vi "Read.vi"(7 "I2C Channel":u8, 8 "Error In":errorcluster, 9 "Range Magnitude (g's)":u16=2, 10 "I2C Slave Address (0x1D)":u8, 11 "LINX Resource in":T1) -> (0 "Error Out":errorcluster, 2 "Acceleration Data (g)":T7, 3 "LINX Resource out":T1)   [LabVIEW 2020, in "LMH-LINX.lvlib" / "MMA8452.lvlib"]
uses:
  MMA8452.lvlib
  Private/Type Defs/LINX Ref.ctl
  Private/Type Defs/Platform.ctl
  Private/Type Defs/Interface.ctl
  Private/Device/Type Defs/LINX Device Config.ctl
  Private/Device/Type Defs/TCP Config.ctl
  Private/Device/Type Defs/Channels.ctl
  Private/Type Defs/Peripherals/I2C/EOF.ctl
  Private/Local IO/LinxI2cWrite.vi
  Utilities/Check Channel.vi
  Private/Utilties/Generate Error.vi
  LMH-LINX.lvlib
  Toolbox/LMH-Toolbox.lvlib
  Private/Device/Device.lvlib
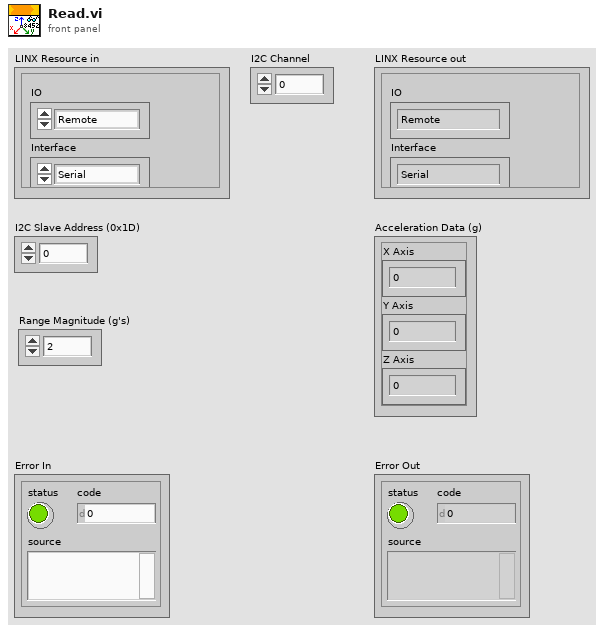
[diagram p1: front panel]
types:
  T1 = typedef "LMH-LINX.lvlib/LINX Ref.ctl" = cluster{"IO":T2, "Interface":T3, "LINX Device Config":T4}
  T2 = typedef "LMH-LINX.lvlib/Platform.ctl" = enum16{"Remote", "Local"}
  T3 = typedef "LMH-LINX.lvlib/Interface.ctl" = enum16{"Serial", "TCP"}
  T4 = typedef "Device.lvlib/LINX Device Config.ctl" = cluster{"Interface":T3, "COM Port":refnum<visa-resource-name>, "TCP Configuration":T5, "Device Family":u8, "Device ID":u8, "Device Name":string, "TCP Ref":refnum<k5>, "Channels":T6}
  T5 = typedef "Device.lvlib/TCP Config.ctl" = cluster{"IP Address":string, "Port":u16}
  T6 = typedef "LMH-LINX.lvlib/Channels.ctl" = cluster{"DI":u8[], "DO":u8[], "AI":u8[], "AO":u8[], "PWM":u8[], "QE":u8[], "UART":u8[], "I2C 2":u8[], "SPI":u8[], "CAN":u8[], "Servo":u8[], "AI Ref (V)":dbl, "AI Resolution (Bits)":u8, "AO Ref (V)":dbl, "AO Resolution (Bits)":u8}
  T7 = cluster{"X Axis":dbl, "Y Axis":dbl, "Z Axis":dbl}
  T8 = typedef "LMH-LINX.lvlib/EOF.ctl" = enum8{"Stop", "Restart", "Restart No Stop", "No Stop"}
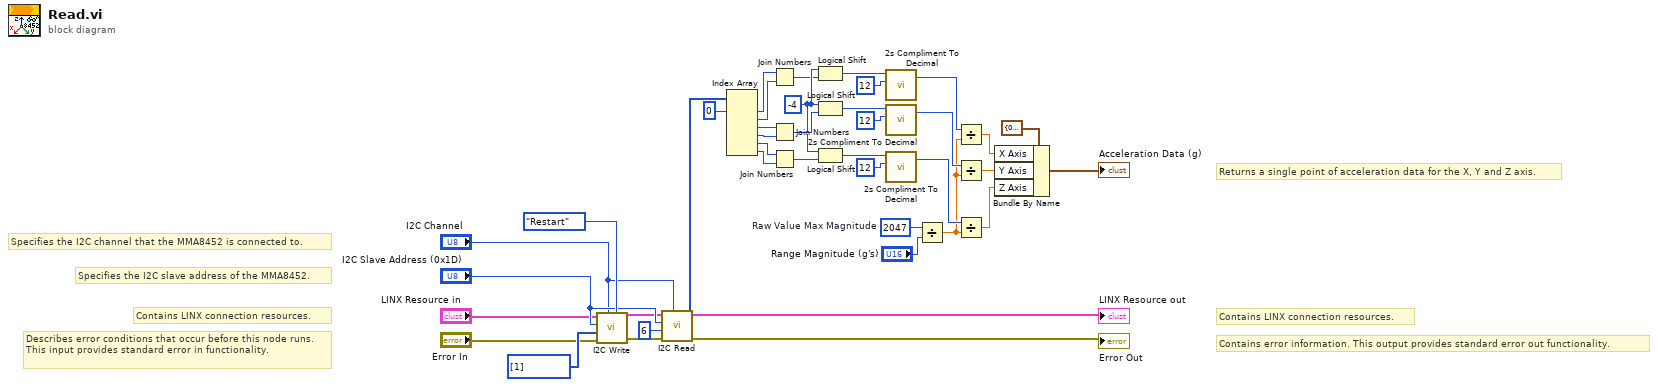
[diagram p0: block diagram]
diagram:
  w36 = i8 -4 ("y")
  w14 = u16 2047  # Raw Value Max Magnitude
  # "Returns a single point of acceleration data for the X, Y and Z axis."
  # "Contains LINX connection resources."
  # "Contains error information. This output provides standard error out functionality."
  # "Specifies the I2C slave address of the MMA8452."
  # "Specifies the I2C channel that the MMA8452 is connected to."
  # "Contains LINX connection resources."
  # "Describes error conditions that occur before this node runs. This input provides standard error in functionality."
  n1 = call "I2C Write.vi"("EOF"=EOF."Restart", "I2C Channel"="I2C Channel", "Error In"="Error In", "Data"=u8[] [1], "I2C Slave Address (0)"="I2C Slave Address (0x1D)", "LINX Resource"="LINX Resource in") -> ("Error Out"=w3:errorcluster, "LINX Resource"=w4:T1)  [unwired: 4 in]
  n2 = call "I2C Read.vi"("I2C Channel"="I2C Channel", "Error In"=w3, "Bytes To Read"=u8 6, "I2C Slave Address (0)"="I2C Slave Address (0x1D)", "LINX Resource"=w4) -> ("Error Out"=→"Error Out":errorcluster, "Data"=w11:u8[], "LINX Resource"=→"LINX Resource out":T1)  [unwired: 4 in]
  n3 = Index Array(array=w11, index #1=0 ("index")) -> (element #1=w21:u8, element #2=w13:u8, element #3=w22:u8, element #4=w23:u8, element #5=w24:u8, element #6=w25:u8)  [unwired: 5 in]
  n4 = Join Numbers(hi=w21, lo=w13) -> ((hi.lo)=w34:u16)
  n5 = Join Numbers(hi=w22, lo=w23) -> ((hi.lo)=w37:u16)
  n6 = Join Numbers(hi=w24, lo=w25) -> ((hi.lo)=w32:u16)
  n7 = Logical Shift(y=w36, x=w34) -> (x << y=w35:u16)
  n8 = Logical Shift(y=w36, x=w37) -> (x << y=w38:u16)
  n9 = Logical Shift(y=w36, x=w32) -> (x << y=w33:u16)
  n10 = call "2s Compliment To Decimal.vi"("Bit Width (8)"=12 ("Width (bits)"), "2s Comp Number"=w35) -> ("Decimal Number"=w31:i32)  [unwired: 3 in]
  n11 = call "2s Compliment To Decimal.vi"("Bit Width (8)"=12 ("Width (bits)"), "2s Comp Number"=w38) -> ("Decimal Number"=w30:i32)  [unwired: 3 in]
  n12 = call "2s Compliment To Decimal.vi"("Bit Width (8)"=12 ("Width (bits)"), "2s Comp Number"=w33) -> ("Decimal Number"=w29:i32)  [unwired: 3 in]
  n13 = Divide(x=w14, y="Range Magnitude (g's)") -> (x/y=w15:dbl)
  n14 = Divide(x=w31, y=w15) -> (x/y=w17:dbl)
  n15 = Divide(x=w30, y=w15) -> (x/y=w18:dbl)
  n16 = Divide(x=w29, y=w15) -> (x/y=w19:dbl)
  n17 = Bundle By Name(cluster=T7 {"X Axis"=0.0, "Y Axis"=0.0, "Z Axis"=0.0} ("Acceleration Data (g)"), "X Axis"=w17, "Y Axis"=w18, "Z Axis"=w19) -> (→"Acceleration Data (g)":T7)
